vi "GF_CheckAgilentInit.vi"(0 "Agilent Control In":T1={"Trig?"=FALSE, "VISA session"="Agilent6034", "Setup to Load"="2", "Timeout (ms)"=40000, "Desired Samp"=enum."1000", "Captured Samp"=11, "Desired Channels"=[{"Chan Index"=enum."Channel1", "Name"="Chan1Test", "Samples"=0}, {"Chan Index"=enum."Channel2", "Name"="Chan2Test", "Samples"=0}, {"Chan Index"=enum."Channel3", "Name"="Chan3Test", "Samples"=0}, {"Chan Index"=enum."Channel4", "Name"="Chan4Test", "Samples"=0}]}) -> (1 "Success":bool, 2 "error out":errorcluster)   [LabVIEW 2020]
uses:
  AgilentControl.ctl
  Channel Config.ctl
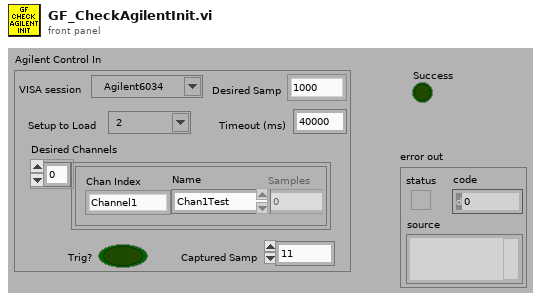
[diagram p1: front panel]
types:
  T1 = typedef "AgilentControl.ctl" = cluster{"Trig?":bool, "VISA session":refnum<visa-resource-name>, "Setup to Load":string, "Timeout (ms)":u32, "Desired Samp":enum32{"100", "250", "500", "1000", "2000", "5000", "10000", "20000", "50000", "100000", "200000", "500000", "1000000", "2000000", "4000000", "8000000"}, "Captured Samp":i32, "Desired Channels":T2[]}
  T2 = typedef "Channel Config.ctl" = cluster{"Chan Index":enum16{"Channel1", "Channel2", "Channel3", "Channel4", "MATH"}, "Name":string, "Samples":i32}
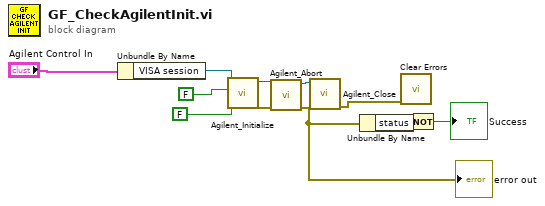
[diagram p0: block diagram]
diagram:
  n1 = Unbundle By Name("Agilent Control In") -> ("VISA session"=w11:refnum<visa-resource-name>)
  n2 = call "Agilent_Initialize.vi"("Reset? (T: Yes)"=FALSE, "ID Query? (T: Yes)"=FALSE, "VISA resource name"=w11) -> ("error out"=w7:errorcluster, "VISA resource name out"=w8:refnum<visa-resource-name>)  [unwired: 7 in]
  n3 = call "Agilent_Abort.vi"("error in (no error)"=w7, "VISA resource name"=w8) -> ("error out"=w4:errorcluster, "VISA resource name out"=w6:refnum<visa-resource-name>)  [unwired: 8 in]
  "error out" <- w4
  n4 = call "Agilent_Close.vi"("VISA resource name"=w6) -> ("error out"=w5:errorcluster)  [unwired: 10 in]
  n5 = Unbundle By Name(w4) -> ("status"=w9:bool)
  n6 = call <vilib>:"Clear Errors.vi"("error in (no error)"=w5) -> ()  [unwired: 5 in, 2 out]
  n7 = Not(x=w9) -> (.not. x?=→"Success":bool)
